vi "Build Command Message.vi"(6 "Command":T1, 8 "error in":errorcluster, 10 "Parameter":dbl, 11 "Kronos in":refnum<class "Kronos.lvclass">) -> (0 "error out":errorcluster, 3 "Kronos out":refnum<class "Kronos.lvclass">)   [LabVIEW 2018, in "Kronos.lvlib" / "Kronos.lvclass"]
uses:
  Kronos.lvclass
  builds/Laser.lvlibp/Custom Controls/Command List.ctl
  Kronos.lvclass/Kronos.ctl
  builds/Laser.lvlibp
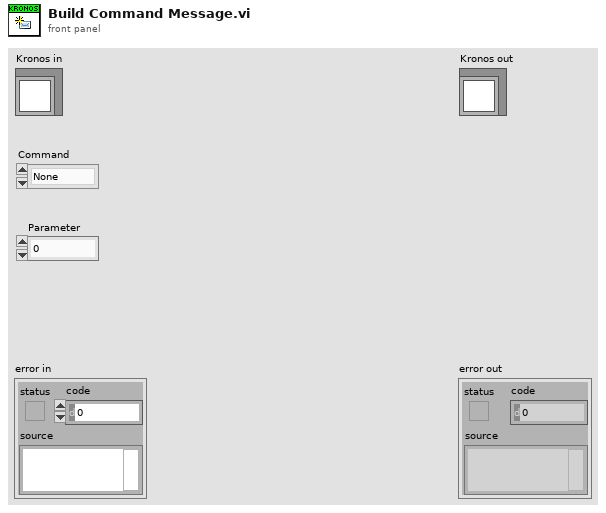
[diagram p1: front panel]
types:
  T1 = typedef "Laser.lvlibp/Command List.ctl" = enum16{"None", "Config?", "Volt?", "ThCase?", "STS?", "Mon?", "Help?", "HB", "Verbose", "Spnt", "Ext", "PRF", "Start", "Stop", "PRF?", "State?", "Status?", "Stat?", "Read HB", "Logon", "Poutmax", "saveconfig", "Reset", "Poutmax?", "PoutCommandMax", "PoutCommandMax?", "FreqMin", "FreqMin?"}
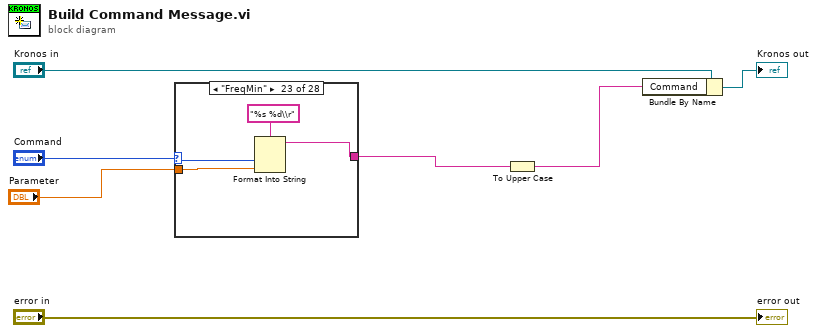
[diagram p0: block diagram]
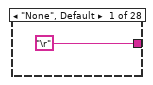
[diagram p2: hidden frame]
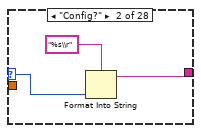
[diagram p3: hidden frame]
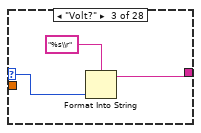
[diagram p4: hidden frame]
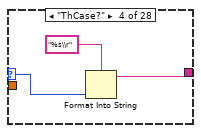
[diagram p5: hidden frame]
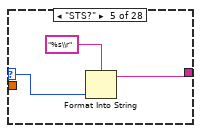
[diagram p6: hidden frame]
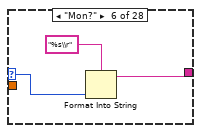
[diagram p7: hidden frame]
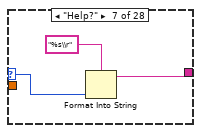
[diagram p8: hidden frame]
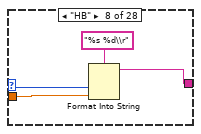
[diagram p9: hidden frame]
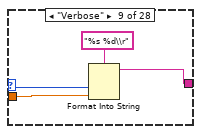
[diagram p10: hidden frame]
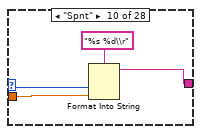
[diagram p11: hidden frame]
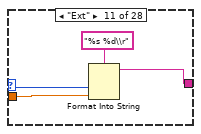
[diagram p12: hidden frame]
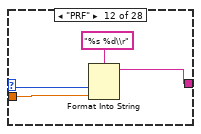
[diagram p13: hidden frame]
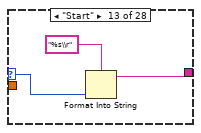
[diagram p14: hidden frame]
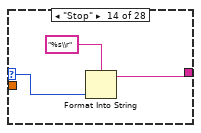
[diagram p15: hidden frame]
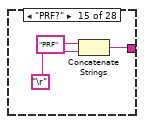
[diagram p16: hidden frame]
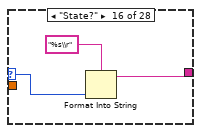
[diagram p17: hidden frame]
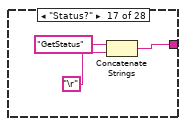
[diagram p18: hidden frame]
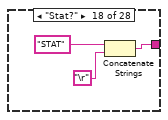
[diagram p19: hidden frame]
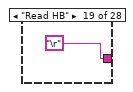
[diagram p20: hidden frame]
diagram:
  n1 = case shown="\"FreqMin\"" "Command" {
    selector: "Command" -> [_ w11 w14 w17 w20 w23 w26 w30 w34 w38 w42 w46 w49 w52 _ w58 _ _ _ w68 w72 w76 w80 w83 w86 _ _ _]
    tunnel: "Parameter" -> [_ _ _ _ _ _ _ w29 w33 w37 w41 w45 _ _ _ _ _ _ _ _ w71 w75 w79 _ _ _ _ _]
    tunnel: ["\r" w9 w12 w15 w18 w21 w24 w27 w31 w35 w39 w43 w47 w50 w55 w56 w60 w63 "\r" w66 w69 w73 w77 w81 w85 w88 w91 w94] -> w2
    frame "None", Default {
    }
    frame "Config?" {
      n2 = Format Into String(format string="%s\\r", w11) -> (resulting string=w9:string)  [unwired: 2 in, 1 out]
    }
    frame "Volt?" {
      n3 = Format Into String(format string="%s\\r", w14) -> (resulting string=w12:string)  [unwired: 2 in, 1 out]
    }
    frame "ThCase?" {
      n4 = Format Into String(format string="%s\\r", w17) -> (resulting string=w15:string)  [unwired: 2 in, 1 out]
    }
    frame "STS?" {
      n5 = Format Into String(format string="%s\\r", w20) -> (resulting string=w18:string)  [unwired: 2 in, 1 out]
    }
    frame "Mon?" {
      n6 = Format Into String(format string="%s\\r", w23) -> (resulting string=w21:string)  [unwired: 2 in, 1 out]
    }
    frame "Help?" {
      n7 = Format Into String(format string="%s\\r", w26) -> (resulting string=w24:string)  [unwired: 2 in, 1 out]
    }
    frame "HB" {
      n8 = Format Into String(format string="%s %d\\r", w30, w29) -> (resulting string=w27:string)  [unwired: 2 in, 1 out]
    }
    frame "Verbose" {
      n9 = Format Into String(format string="%s %d\\r", w34, w33) -> (resulting string=w31:string)  [unwired: 2 in, 1 out]
    }
    frame "Spnt" {
      n10 = Format Into String(format string="%s %d\\r", w38, w37) -> (resulting string=w35:string)  [unwired: 2 in, 1 out]
    }
    frame "Ext" {
      n11 = Format Into String(format string="%s %d\\r", w42, w41) -> (resulting string=w39:string)  [unwired: 2 in, 1 out]
    }
    frame "PRF" {
      n12 = Format Into String(format string="%s %d\\r", w46, w45) -> (resulting string=w43:string)  [unwired: 2 in, 1 out]
    }
    frame "Start" {
      n13 = Format Into String(format string="%s\\r", w49) -> (resulting string=w47:string)  [unwired: 2 in, 1 out]
    }
    frame "Stop" {
      n14 = Format Into String(format string="%s\\r", w52) -> (resulting string=w50:string)  [unwired: 2 in, 1 out]
    }
    frame "PRF?" {
      n15 = Concatenate Strings("PRF", "\r") -> (w55:string)
    }
    frame "State?" {
      n16 = Format Into String(format string="%s\\r", w58) -> (resulting string=w56:string)  [unwired: 2 in, 1 out]
    }
    frame "Status?" {
      n17 = Concatenate Strings("GetStatus", "\r") -> (w60:string)
    }
    frame "Stat?" {
      n18 = Concatenate Strings("STAT", "\r") -> (w63:string)
    }
    frame "Read HB" {
    }
    frame "Logon" {
      n19 = Format Into String(format string="%s pop090\\r", w68) -> (resulting string=w66:string)  [unwired: 2 in, 1 out]
    }
    frame "Poutmax" {
      n20 = Format Into String(format string="%s %d\\r", w72, w71) -> (resulting string=w69:string)  [unwired: 2 in, 1 out]
    }
    frame "PoutCommandMax" {
      n21 = Format Into String(format string="%s %d\\r", w76, w75) -> (resulting string=w73:string)  [unwired: 2 in, 1 out]
    }
    frame "FreqMin" {
      n22 = Format Into String(format string="%s %d\\r", w80, w79) -> (resulting string=w77:string)  [unwired: 2 in, 1 out]
    }
    frame "saveconfig" {
      n23 = Format Into String(format string="%s\\r", w83) -> (resulting string=w81:string)  [unwired: 2 in, 1 out]
    }
    frame "Reset" {
      n24 = Format Into String(format string="%s 1\\r", w86) -> (resulting string=w85:string)  [unwired: 2 in, 1 out]
    }
    frame "Poutmax?" {
      n25 = Concatenate Strings("Poutmax", "\r") -> (w88:string)
    }
    frame "PoutCommandMax?" {
      n26 = Concatenate Strings("Poutcommandmax", "\r") -> (w91:string)
    }
    frame "FreqMin?" {
      n27 = Concatenate Strings("FREQMIN", "\r") -> (w94:string)
    }
  }
  n28 = To Upper Case(1:w2) -> (0:w1:string)
  n29 = Bundle By Name(cluster="Kronos in", "Command"=w1) -> (→"Kronos out":refnum<class "Kronos.lvclass">)
  "error out" <- "error in"
